vi "readDataFromMachine.vi"(0 "VISA resource name":refnum<visa-resource-name>, 6 "error in (no error)":errorcluster, 10 "file (use dialog)":path) -> (12 "Frequency":string, 14 "VX":string, 16 "VY":string, 18 "VR":string, 20 "VISA resource name out":refnum<visa-resource-name>, 21 "Phase":string, 22 "refnum out":refnum<file>, 26 "error out":errorcluster)   [LabVIEW 2012]
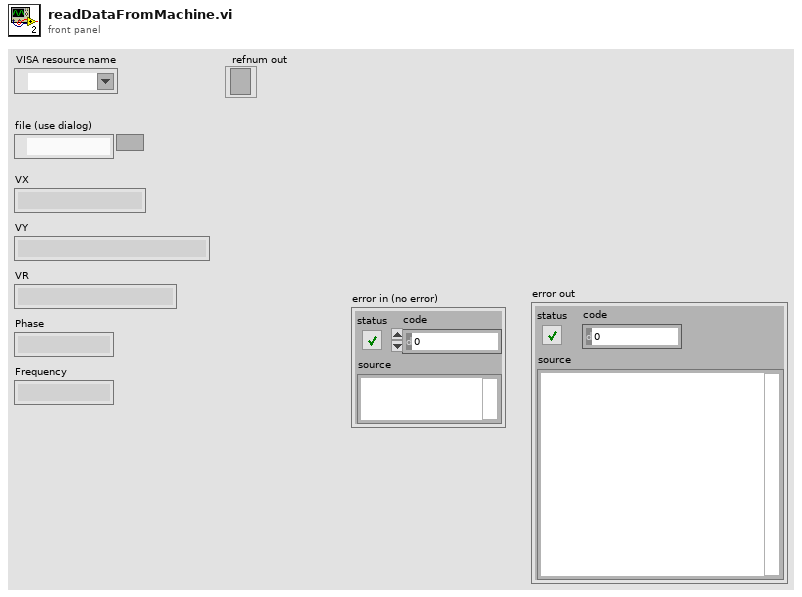
[diagram p1: front panel]
types:
  T1 = enum16{"open", "replace", "create", "open or create", "replace or create", "replace or create with confirmation"}
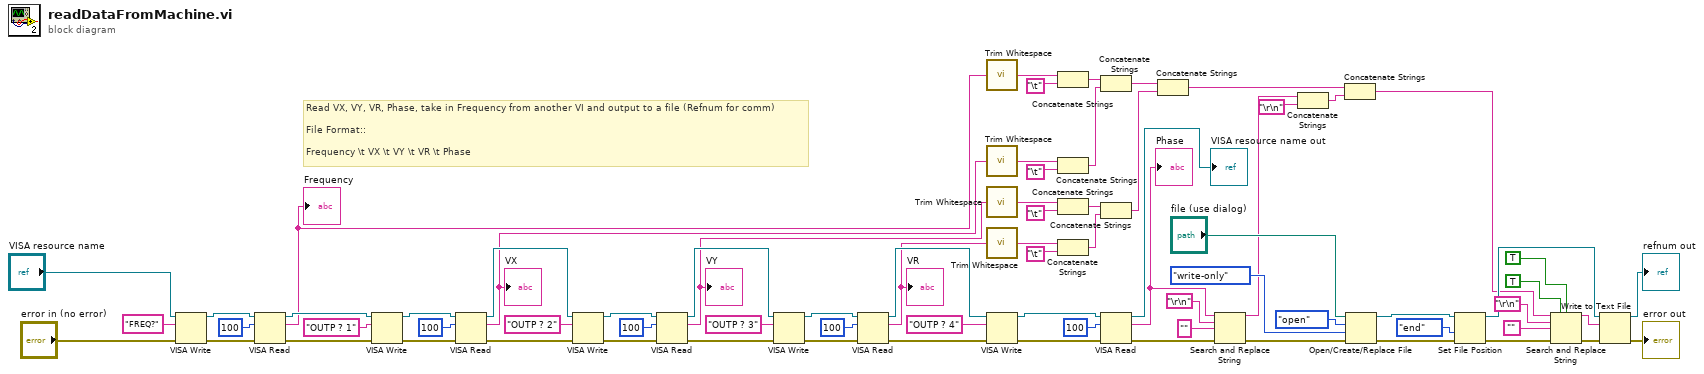
[diagram p0: block diagram]
diagram:
  # "Read VX, VY, VR, Phase, take in Frequency from another VI and output to a file (Refnum for comm)\n\nFile Format::\n\nFrequency \\t VX \\t VY \\t VR \\t Phase"
  n1 = VISA Write(VISA resource name="VISA resource name", write buffer="FREQ?", error in (no error)="error in (no error)") -> (VISA resource name out=w71:refnum<visa-resource-name>, error out=w70:errorcluster)  [unwired: 1 out]
  n2 = VISA Read(VISA resource name=w71, byte count=u32 100, error in (no error)=w70) -> (VISA resource name out=w30:refnum<visa-resource-name>, read buffer=w11:string, error out=w31:errorcluster)  [unwired: 1 out]
  "Frequency" <- w11
  n3 = VISA Write(VISA resource name=w30, write buffer="OUTP ? 1", error in (no error)=w31) -> (VISA resource name out=w41:refnum<visa-resource-name>, error out=w64:errorcluster)  [unwired: 1 out]
  n4 = VISA Read(VISA resource name=w41, byte count=u32 100, error in (no error)=w64) -> (VISA resource name out=w42:refnum<visa-resource-name>, read buffer=w8:string, error out=w9:errorcluster)  [unwired: 1 out]
  "VX" <- w8
  n5 = VISA Write(VISA resource name=w42, write buffer="OUTP ? 2", error in (no error)=w9) -> (VISA resource name out=w63:refnum<visa-resource-name>, error out=w40:errorcluster)  [unwired: 1 out]
  n6 = VISA Read(VISA resource name=w63, byte count=u32 100, error in (no error)=w40) -> (VISA resource name out=w57:refnum<visa-resource-name>, read buffer=w5:string, error out=w6:errorcluster)  [unwired: 1 out]
  "VY" <- w5
  n7 = VISA Write(VISA resource name=w57, write buffer="OUTP ? 3", error in (no error)=w6) -> (VISA resource name out=w62:refnum<visa-resource-name>, error out=w61:errorcluster)  [unwired: 1 out]
  n8 = VISA Read(VISA resource name=w62, byte count=u32 100, error in (no error)=w61) -> (VISA resource name out=w58:refnum<visa-resource-name>, read buffer=w1:string, error out=w2:errorcluster)  [unwired: 1 out]
  "VR" <- w1
  n9 = call <vilib>:"Trim Whitespace.vi"("string"=w11) -> ("trimmed string"=w10:string)  [unwired: 1 in]
  n10 = call <vilib>:"Trim Whitespace.vi"("string"=w8) -> ("trimmed string"=w7:string)  [unwired: 1 in]
  n11 = call <vilib>:"Trim Whitespace.vi"("string"=w5) -> ("trimmed string"=w4:string)  [unwired: 1 in]
  n12 = call <vilib>:"Trim Whitespace.vi"("string"=w1) -> ("trimmed string"=w3:string)  [unwired: 1 in]
  n13 = VISA Write(VISA resource name=w58, write buffer="OUTP ? 4", error in (no error)=w2) -> (VISA resource name out=w59:refnum<visa-resource-name>, error out=w60:errorcluster)  [unwired: 1 out]
  n14 = Concatenate Strings(w10, "\t") -> (w51:string)
  n15 = Concatenate Strings(w7, "\t") -> (w50:string)
  n16 = Concatenate Strings(w4, "\t") -> (w49:string)
  n17 = Concatenate Strings(w3, "\t") -> (w48:string)
  n18 = Concatenate Strings(w51, w50) -> (w47:string)
  n19 = Concatenate Strings(w49, w48) -> (w46:string)
  n20 = VISA Read(VISA resource name=w59, byte count=u32 100, error in (no error)=w60) -> (VISA resource name out=→"VISA resource name out":refnum<visa-resource-name>, read buffer=w15:string, error out=w13:errorcluster)  [unwired: 1 out]
  "Phase" <- w15
  n21 = Concatenate Strings(w47, w46) -> (w45:string)
  n22 = Search and Replace String(input string=w15, search string="\r\n", replace string="" ("replace string (\"\")"), error in=w13) -> (result string=w14:string, error out=w12:errorcluster)  [unwired: 4 in, 2 out]
  n23 = Concatenate Strings(w14, "\r\n") -> (w44:string)
  n24 = Concatenate Strings(w45, w44) -> (w25:string)
  n25 = Open/Create/Replace File(file path (use dialog)="file (use dialog)", error in=w12, operation (0:open)=T1."open", access (0:read/write)=enum16{"read/write", "read-only", "write-only"}."write-only") -> (refnum out=w29:refnum<file>, error out=w26:errorcluster)  [unwired: 2 in, 1 out]
  n26 = Set File Position(refnum=w29, from (0:start)=enum16{"start", "end", "current"}."end", error in=w26) -> (refnum out=w28:refnum<file>, error out=w21:errorcluster)  [unwired: 1 in]
  n27 = Search and Replace String(replace all?=TRUE ("replace all? (F)"), case sensitive?=TRUE ("ignore case? (F)"), input string=w25, search string="\r\n", replace string="", error in=w21) -> (result string=w24:string, error out=w20:errorcluster)  [unwired: 2 in, 2 out]
  n28 = Write to Text File(file (use dialog)=w28, text=w24, error in=w20) -> (refnum out=→"refnum out":refnum<file>, error out=→"error out":errorcluster)  [unwired: 1 in, 1 out]
